vi "Wave generator.vi"   [LabVIEW 2014]
uses:
  <vilib>/Platform/TimedLoop/XDataNode/timing_clust.ctl
  <vilib>/Platform/TimedLoop/XDataNode/nitl_modes.ctl
  <vilib>/Platform/TimedLoop/XDataNode/wakeup.ctl
  <vilib>/rvi/Emulation/niFpgaSctlEmulationGetInTimedLoop.vi
  <vilib>/rvi/Emulation/niFpgaEmulationReportErrorSimple.vi
  <vilib>/rvi/Emulation/niFpgaGetClockAttributes.vi
  <vilib>/rvi/Emulation/niFpgaCriticalErrorInLSC.vi
  <vilib>/rvi/Memory/Memory_Emulation/nirvimemoryFastEmulation.vi
  <vilib>/rvi/Memory/Memory_Emulation/nirvimemoryEmulation.vi
  <vilib>/rvi/Emulation/niFpgaEmulationIsFPGAContextNoSignature.vi
  <vilib>/rvi/DataTransferAndStorage/Container/Common/niFpgaContainerGetUniqueNameForEmu.vi
  <vilib>/rvi/Emulation/niFpgaProcessEmulError.vi
  <vilib>/rvi/errors/nirviReportUnexpectedCaseInternalError (U32).vi
  <vilib>/rvi/eio/common/nirviEmuTemplateMethod_errors.vi
  <vilib>/Platform/TimedLoop/XDataNode/XDataNode.xnode
  <vilib>/rvi/DataTransferAndStorage/Container/XNode/niFpgaContainer.xnode
  <vilib>/eio/EIONode/EIONode.xnode
  <vilib>/Platform/TimedLoop/XDataNode/XDNodeRunTimeDep.lvlib
types:
  T1 = typedef "XDNodeRunTimeDep.lvlib/timing_clust.ctl" = cluster{"Expected End [f-1]":u64, "Actual End [f-1]":u64, "Finished Late? [f-1]":bool, "Expected End [i-1]":u64, "Actual End [i-1]":u64, "Finished Late? [i-1]":bool, "Expected Start [i]":u64, "Actual Start [i]":u64, "Expected Start [f]":u64, "Actual Start [f]":u64, "Source Name":string, "Structure Name":string, "Period":i64, "Deadline":i64, "Offset":i64, "Start":i64, "Priority":i32, "Timeout":i32, "Mode":T2, "Wakeup Reason":T3, "Error":errorcluster, "Source Type":string, "Secondary Source Type":string, "Global End Time":u64, "Global Start Time":u64, "Frame Duration":u64, "Iteration Duration":u64, "Assigned CPU":i32, "I/O Scan Engine Mode":u32}
  T2 = typedef "XDNodeRunTimeDep.lvlib/nitl_modes.ctl" = enum32{"No Change", "Process missed periods, maintain original phase", "Discard missed periods, maintain original phase", "Process missed periods, ignore original phase", "Discard missed periods, ignore original phase"}
  T3 = typedef "XDNodeRunTimeDep.lvlib/wakeup.ctl" = enum32{"Normal", "Aborted", "Asynchronous wakeup", "Timing source error", "Timed loop error", "Timeout"}
  T4 = cluster{"Boolean array[0]":bool, "Boolean array[1]":bool, "Boolean array[2]":bool, "Boolean array[3]":bool, "Boolean array[4]":bool, "Boolean array[5]":bool, "Boolean array[6]":bool, "Boolean array[7]":bool, "Boolean array[8]":bool, "Boolean array[9]":bool, "Boolean array[10]":bool, "Boolean array[11]":bool}
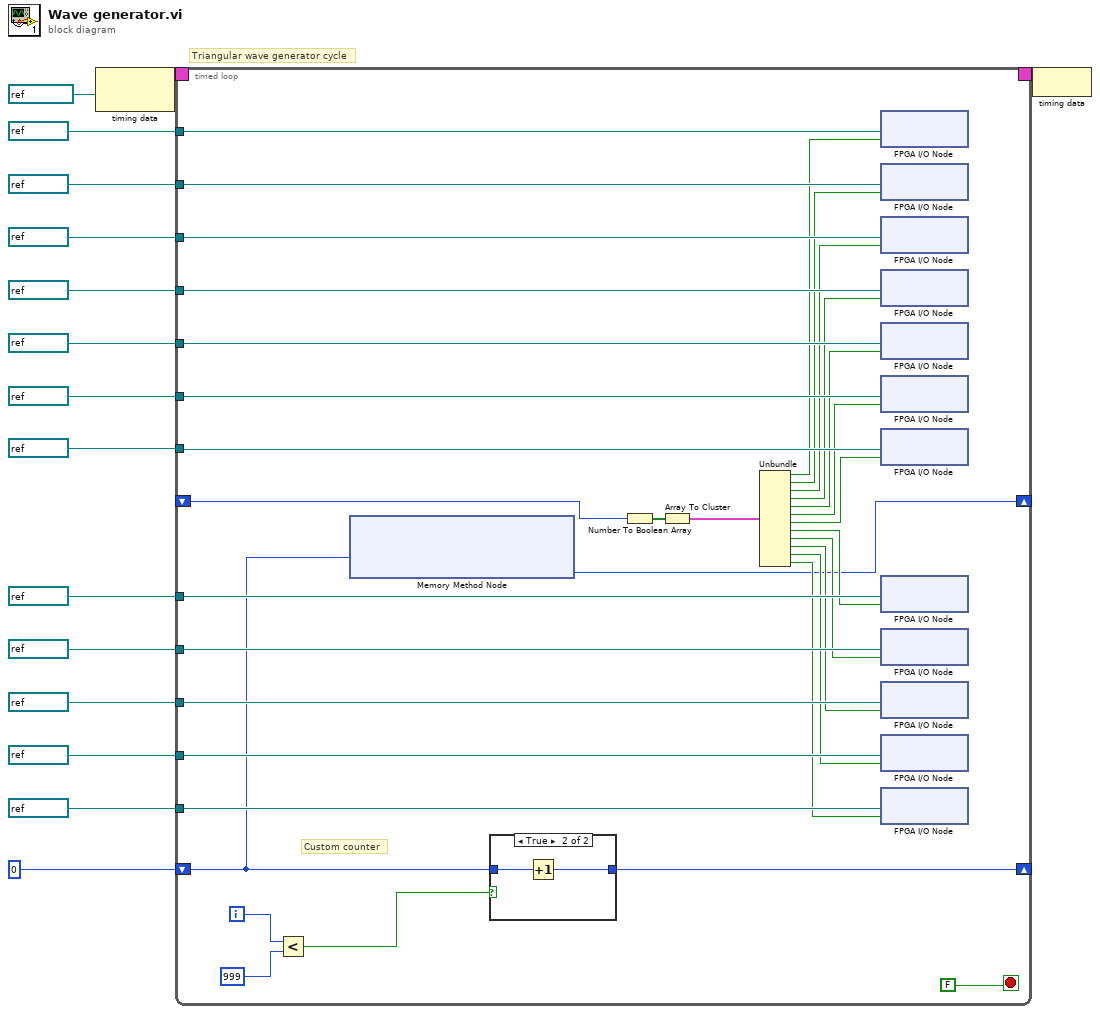
[diagram p0: block diagram]
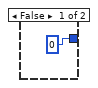
[diagram p2: hidden frame]
diagram:
  # "Triangular wave generator cycle"
  n1 = node-c288(refnum<k21> "50MHz" ("Source Name")) -> (w16:T1)
  n2 = timed-loop {
    timing: w16 -> [_]
    timing-out: [_] -> w15
    shift-right: [w46] -> _
    shift-left: u32 0 -> [w19]
    tunnel: refnum<k21> "DIO12" ("FPGA I/O In") -> [w43]
    tunnel: refnum<k21> "DIO13" ("FPGA I/O In") -> [w42]
    tunnel: refnum<k21> "DIO14" ("FPGA I/O In") -> [w41]
    tunnel: refnum<k21> "DIO15" ("FPGA I/O In") -> [w40]
    tunnel: refnum<k21> "DIO16" ("FPGA I/O In") -> [w39]
    tunnel: refnum<k21> "DIO17" ("FPGA I/O In") -> [w38]
    tunnel: refnum<k21> "DIO18" ("FPGA I/O In") -> [w37]
    tunnel: refnum<k21> "DIO19" ("FPGA I/O In") -> [w36]
    tunnel: refnum<k21> "DIO20" ("FPGA I/O In") -> [w35]
    tunnel: refnum<k21> "DIO21" ("FPGA I/O In") -> [w34]
    tunnel: refnum<k21> "DIO22" ("FPGA I/O In") -> [w33]
    tunnel: refnum<k21> "DIO23" ("FPGA I/O In") -> [w32]
    shift-right: [w18] -> _
    shift-left: _ -> [w17]
    i -> [w48]
    stop <- FALSE stop-if-true
    # "Custom counter"
    n3 = Less?(x=w48, y=999) -> (x < y?=w49:bool)
    n4 = xnode ("Memory Method Node")("Address A"=w19) -> ("Data A"=w18:i16)  [unwired: 1 in, 1 out]
    n5 = case shown="True" w49 {
      tunnel: w19 -> [_ w53]
      tunnel: [u32 0 w52] -> w46
      frame False {
      }
      frame True {
        n6 = Increment(x=w53) -> (x+1=w52:u32)
      }
    }
    n7 = Number To Boolean Array(number=w17) -> (Boolean array=w45:bool[])
    n8 = Array To Cluster(array=w45) -> (cluster=w44:T4)
    n9 = Unbundle(w44) -> ("Boolean array[0]"=w31:bool, "Boolean array[1]"=w30:bool, "Boolean array[2]"=w29:bool, "Boolean array[3]"=w28:bool, "Boolean array[4]"=w27:bool, "Boolean array[5]"=w26:bool, "Boolean array[6]"=w25:bool, "Boolean array[7]"=w24:bool, "Boolean array[8]"=w23:bool, "Boolean array[9]"=w22:bool, "Boolean array[10]"=w21:bool, "Boolean array[11]"=w20:bool)
    n10 = xnode "FPGA I/O Node"("I/O Item"=w31, "FPGA I/O In"=w43) -> ()  [unwired: 1 out]
    n11 = xnode "FPGA I/O Node"("I/O Item"=w30, "FPGA I/O In"=w42) -> ()  [unwired: 1 out]
    n12 = xnode "FPGA I/O Node"("I/O Item"=w29, "FPGA I/O In"=w41) -> ()  [unwired: 1 out]
    n13 = xnode "FPGA I/O Node"("I/O Item"=w28, "FPGA I/O In"=w40) -> ()  [unwired: 1 out]
    n14 = xnode "FPGA I/O Node"("I/O Item"=w27, "FPGA I/O In"=w39) -> ()  [unwired: 1 out]
    n15 = xnode "FPGA I/O Node"("I/O Item"=w26, "FPGA I/O In"=w38) -> ()  [unwired: 1 out]
    n16 = xnode "FPGA I/O Node"("I/O Item"=w25, "FPGA I/O In"=w37) -> ()  [unwired: 1 out]
    n17 = xnode "FPGA I/O Node"("I/O Item"=w24, "FPGA I/O In"=w36) -> ()  [unwired: 1 out]
    n18 = xnode "FPGA I/O Node"("I/O Item"=w23, "FPGA I/O In"=w35) -> ()  [unwired: 1 out]
    n19 = xnode "FPGA I/O Node"("I/O Item"=w22, "FPGA I/O In"=w34) -> ()  [unwired: 1 out]
    n20 = xnode "FPGA I/O Node"("I/O Item"=w21, "FPGA I/O In"=w33) -> ()  [unwired: 1 out]
    n21 = xnode "FPGA I/O Node"("I/O Item"=w20, "FPGA I/O In"=w32) -> ()  [unwired: 1 out]
  }
  n22 = node-c288(w15) -> ()
